vi "LIA Debugging Slow FPGA.vi"() -> ()   [LabVIEW 2018]
uses:
  <vilib>/eio/EIONode/EIONode.xnode
  <vilib>/rvi/eio/common/nirviEmuTemplateMethod_errors.vi
  <vilib>/Platform/TimedLoop/XDataNode/wakeup.ctl
  <vilib>/Platform/TimedLoop/XDataNode/XDNodeRunTimeDep.lvlib
  <vilib>/Platform/TimedLoop/XDataNode/nitl_modes.ctl
  <vilib>/Platform/TimedLoop/XDataNode/timing_clust.ctl
  <vilib>/Platform/TimedLoop/XDataNode/XDataNode.xnode
  <instrlib>/_niInstr/Basic Elements/v1/FPGA/niInstr Basic Elements v1 FPGA.lvlib
  <instrlib>/_niInstr/DSP/v1/Shared/Public/IQ Data.ctl
  <instrlib>/_niInstr/DSP/v1/Shared/niInstr DSP v1 Shared.lvlib
  <instrlib>/_niInstr/DSP/v1/FPGA/niInstr DSP v1 FPGA.lvlib
  <instrlib>/_niInstr/DSP/v1/Xnodes/Public/Frequency Shift/niInstr DSP v1 Frequency Shift FPGA.xnode
  Shared/_NI PLL IP/FPGA/NI PLL IP FPGA.lvlib
  <vilib>/rvi/FXPMathLib/FxpMul/XNode/nifxpmath_Multiplier.xnode
  <vilib>/rvi/FXPMathLib/FxpAdd/XNode/nifxpmath_Add.xnode
  <instrlib>/_niInstr/DSP/v1/FPGA/Public/Sub VIs/Frequency Shift/Frequency Shift - 2 spc.vi
  Shared/lib/fpga/Lock-In Amplifier Example FPGA.lvlib
  <instrlib>/_niInstr/Streaming/v1/Common/Stream State.ctl
  <instrlib>/_niInstr/Streaming/v1/Common/niInstr Streaming v1 Common.lvlib
  <userlib>/_NI Noise Generation IP/FPGA/NI Noise Generation IP FPGA v2.lvlib
  <vilib>/rvi/FXPMathLib/sim/FxpSim.dll
  <instrlib>/_niInstr/DSP/v1/FPGA/Public/Sub VIs/Fractional Decimator/Fractional Decimator - 1 spc - 2x oc.vi
  <userlib>/_NI Noise Generation IP/FPGA/Public/Low Level/AWGN FXP23x2.vi
  <instrlib>/_niInstr/Data Trigger/v1/Shared/Public/Edge Configuration Trigger Slope.ctl
  <instrlib>/_niInstr/Data Trigger/v1/Shared/niInstr Data Trigger v1 Shared.lvlib
  <instrlib>/_niInstr/Data Trigger/v1/Shared/Public/Edge Configuration FXP(+-,18,1).ctl
  Shared/SOS/Controls/IIR_Coeffs.ctl
panel:
  out "lock-in.fir overflow? 0":bool
  out "lock-in.prefilter fir overflow? 0":bool
  out "lock-in.fs overflow? 0":bool
  in  "lock-in.iir config prefilter 0":T1
  in  "lock-in.iir prefilter decmation 0":fxp<+,4,4>
  out "stream.overflow? 0":bool
  in  "all.clear overflow 0":bool
  in  "lock-in.fir fs prefilter 0":fxp<+,48,1>
  in  "lock-in.prefilter 0":enum16{"1x2SOS", "None", "FIR"}(ring)
  in  "lock-in.iir enable0 0":bool
  in  "lock-in.iir decimation0 0":fxp<+,4,4> format="%#_3g"
  in  "lock-in.iir config0 0":T1={"b0"=0.015777587890625, "b1"=-0.030517578125, "-a1"=1.9578399658203125, "-a2"=-0.9589080810546875}
  in  "nco.enable 0":bool=TRUE
  in  "nco.reset 0":bool
  in  "nco.frequency 0":fxp<+/-,48,0>
  in  "lock-in.fir0 fs 0":fxp<+,48,1>
  in  "lock-in.decimator0 0":enum16{"None", "CIC", "FIR", "2x4HB", "2x4SOS"}(ring)
  in  "dpll.reset 1":bool
  in  "dpll.enable 1":bool
  in  "dpll.q 1":fxp<+/-,48,0>
  in  "dpll.m 1":i8
  in  "dpll.config 1":T2
  out "dpll.vco output 1":fxp<+/-,48,0>
  in  "dpll.channel 1":i32
  in  "dpll.channel 0":i32
  out "dpll.vco output 0":fxp<+/-,48,0>
  in  "dpll.config 0":T2
  in  "dpll.m 0":i8
  in  "dpll.q 0":fxp<+/-,48,0>
  in  "dpll.enable 0":bool
  in  "dpll.reset 0":bool
  in  "lock-in.enable 3":bool
  in  "lock-in.enable 2":bool
  in  "lock-in.enable 1":bool
  in  "lock-in.carrier 3":fxp<+/-,48,0>
  in  "lock-in.carrier 2":fxp<+/-,48,0>
  in  "lock-in.enable 0":bool
  in  "lock-in.channel select 3":i32
  in  "lock-in.carrier select 3":i32
  in  "lock-in.cic config valid 3":bool
  in  "lock-in.cic config 3":cluster{"factor":fxp<+,16,16>, "shift":i16}
  in  "lock-in.reset 3":bool
  out "stream.state 3":T4 caption="stream.state 0"
  out "stream.samples transferred 3":u64 caption="stream.samples transferred 0"
  out "stream.metadata 3":u64 caption="stream.metadata 0"
  in  "stream.num samples 3":u64 caption="stream.num samples 0"
  in  "stream.request state 3":T4 caption="stream.request state 0"
  in  "lock-in.channel select 2":i32
  in  "lock-in.carrier select 2":i32
  in  "lock-in.cic config valid 2":bool
  in  "lock-in.cic config 2":cluster{"factor":fxp<+,16,16>, "shift":i16}
  in  "lock-in.reset 2":bool
  out "stream.state 2":T4 caption="stream.state 0"
  out "stream.samples transferred 2":u64 caption="stream.samples transferred 0"
  out "stream.metadata 2":u64 caption="stream.metadata 0"
  in  "stream.num samples 2":u64 caption="stream.num samples 0"
  in  "stream.request state 2":T4 caption="stream.request state 0"
  out "pll.vco output 0":fxp<+/-,48,0>
  out "pll.vco output 1":fxp<+/-,48,0>
  out "stream.metadata 4":u64 caption="stream.metadata 0"
  out "stream.samples transferred 4":u64 caption="stream.samples transferred 0"
  out "stream.state 4":T4 caption="stream.state 0"
  in  "stream.request state 4":T4 caption="stream.request state 0"
  in  "stream.num samples 4":u64 caption="stream.num samples 0"
  in  "preview.channel select":i32
  in  "ao.reset 3":bool
  in  "ao.carrier 2":fxp<+/-,48,0>=0.010000000000001563
  in  "ao.level 2":fxp<+/-,18,1>
  in  "ao.reset 2":bool
  in  "ao.carrier 1":fxp<+/-,48,0>=0.010000000000001563
  in  "ao.level 1":fxp<+/-,18,1>
  in  "ao.reset 1":bool
  in  "ao.reset 0":bool
  in  "ao.carrier 0":fxp<+/-,48,0>=0.010000000000001563
  in  "ao.level 0":fxp<+/-,18,1>
  in  "lock-in.channel select 1":i32
  in  "lock-in.channel select 0":i32
  in  "stream.request state 1":T4 caption="stream.request state 0"
  in  "stream.num samples 1":u64 caption="stream.num samples 0"
  out "stream.metadata 1":u64 caption="stream.metadata 0"
  out "stream.samples transferred 1":u64 caption="stream.samples transferred 0"
  out "stream.state 1":T4 caption="stream.state 0"
  in  "lock-in.reset 1":bool
  in  "lock-in.cic config 1":cluster{"factor":fxp<+,16,16>, "shift":i16}
  in  "lock-in.cic config valid 1":bool
  in  "lock-in.carrier select 1":i32
  in  "lock-in.carrier select 0":i32
  in  "lock-in.cic config valid 0":bool
  in  "lock-in.cic config 0":cluster{"factor":fxp<+,16,16>, "shift":i16}
  in  "lock-in.reset 0":bool
  in  "lock-in.carrier 1":fxp<+/-,48,0>
  in  "lock-in.carrier 0":fxp<+/-,48,0>
  in  "ao.level 3":fxp<+/-,18,1>
  in  "pll.channel 1":i32
  in  "pll.reset 1":bool
  in  "pll.enable 1":bool
  in  "pll.config 1":T5={"quiescent frequency"=0.10000000000000142, "compensation"=0.0, "psd gain"=-18, "loop filter"={"order"=4, "cutoff"=6}}
  in  "pll.channel 0":i32
  in  "ao.noise gain 3":fxp<+,18,1>=0.01000213623046875
  in  "ao.carrier 3":fxp<+/-,48,0>=0.010000000000001563
  in  "ao.noise seeds 3":fxp<+,23,23>[](array[numeric])=[1.0, 12323.0]
  in  "pll.reset 0":bool
  in  "pll.enable 0":bool
  in  "stream.request state 0":T4
  in  "stream.num samples 0":u64
  out "stream.metadata 0":u64
  out "stream.samples transferred 0":u64
  out "stream.state 0":T4
  in  "pll.config 0":T5={"quiescent frequency"=0.10000000000000142, "compensation"=0.0, "psd gain"=-18, "loop filter"={"order"=4, "cutoff"=6}}
  out "IO Module\\InitDone":bool
  out "IO Module\\User Error":u32
  in  "IO Module\\User Command":u32
  in  "IO Module\\User Command Valid":bool
  out "IO Module\\User Command Ready":bool
  in  "IO Module\\User Command Arg 0":u32
  in  "IO Module\\User Command Arg 1":u32
  out "IO Module\\User Command Error":u16
  out "IO Module\\User Command Return":u32
  out "IO Module\\User Command Return Valid":bool
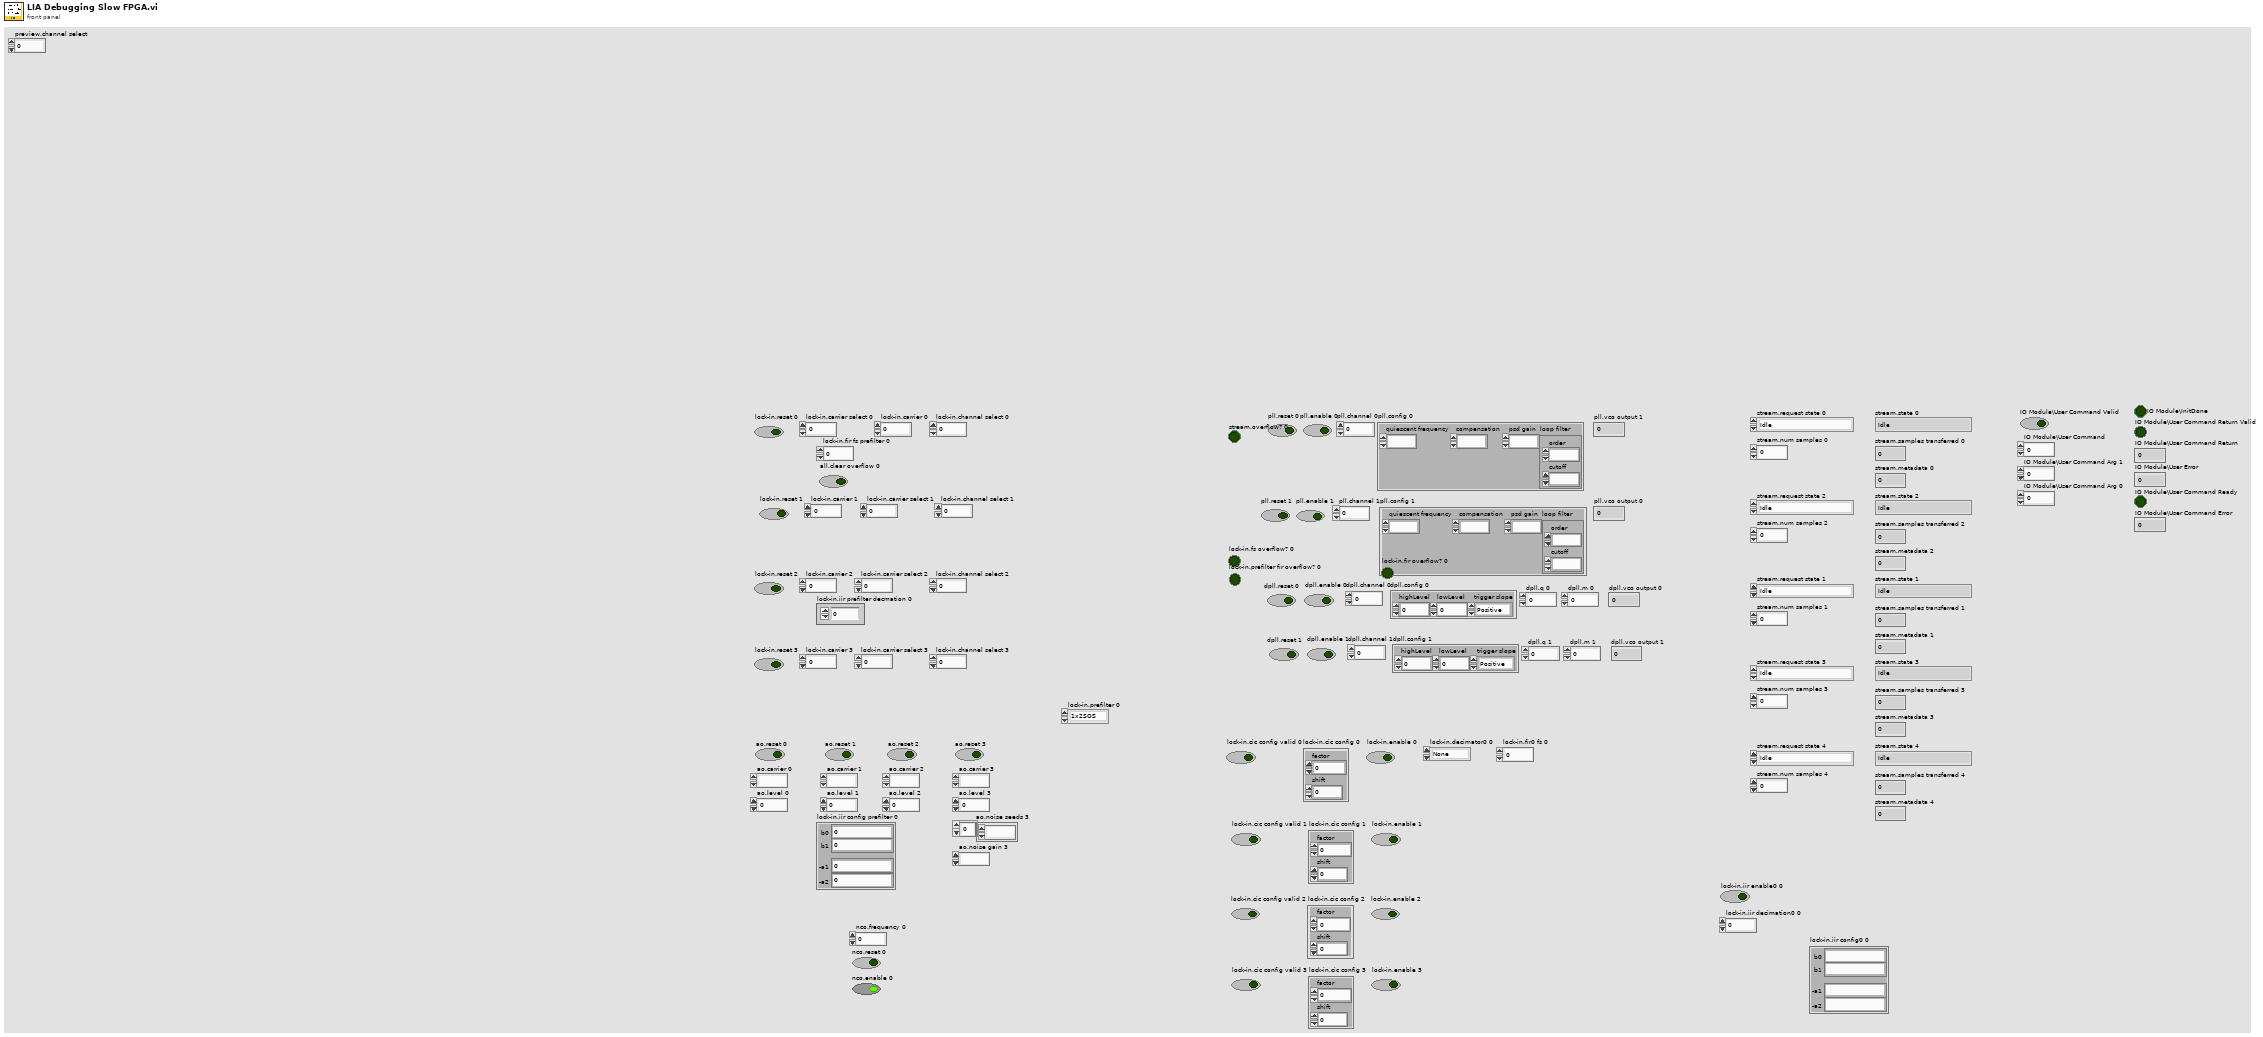
[diagram p1: front panel]
types:
  T1 = typedef "IIR_Coeffs.ctl" = cluster{"b0":fxp<+/-,18,2>, "b1":fxp<+/-,18,2>, "-a1":fxp<+/-,18,2>, "-a2":fxp<+/-,18,2>}
  T2 = typedef "niInstr Data Trigger v1 Shared.lvlib/Edge Configuration FXP(+-,18,1).ctl" = cluster{"highLevel":fxp<+/-,18,1>, "lowLevel":fxp<+/-,18,1>, "trigger slope":T3}
  T3 = typedef "niInstr Data Trigger v1 Shared.lvlib/Edge Configuration Trigger Slope.ctl" = enum8{"Positive", "Negative"}
  T4 = typedef "niInstr Streaming v1 Common.lvlib/Stream State.ctl" = enum8{"Idle", "Finite Transfer", "Continuous", "Done", "Error", "Not Ready", "Cancel"}
  T5 = cluster{"quiescent frequency":fxp<+/-,48,0>, "compensation":fxp<+/-,18,3>, "psd gain":i16, "loop filter":cluster{"order":i32, "cutoff":i8}}
  T6 = typedef "XDNodeRunTimeDep.lvlib/timing_clust.ctl" = cluster{"Expected End [f-1]":u64, "Actual End [f-1]":u64, "Finished Late? [f-1]":bool, "Expected End [i-1]":u64, "Actual End [i-1]":u64, "Finished Late? [i-1]":bool, "Expected Start [i]":u64, "Actual Start [i]":u64, "Expected Start [f]":u64, "Actual Start [f]":u64, "Source Name":string, "Structure Name":string, "Period":i64, "Deadline":i64, "Offset":i64, "Start":i64, "Priority":i32, "Timeout":i32, "Mode":T7, "Wakeup Reason":T8, "Error":errorcluster, "Source Type":string, "Secondary Source Type":string, "Global End Time":u64, "Global Start Time":u64, "Frame Duration":u64, "Iteration Duration":u64, "Assigned CPU":i32, "I/O Scan Engine Mode":u32}
  T7 = typedef "XDNodeRunTimeDep.lvlib/nitl_modes.ctl" = enum32{"No Change", "Process missed periods, maintain original phase", "Discard missed periods, maintain original phase", "Process missed periods, ignore original phase", "Discard missed periods, ignore original phase"}
  T8 = typedef "XDNodeRunTimeDep.lvlib/wakeup.ctl" = enum32{"Normal", "Aborted", "Asynchronous wakeup", "Timing source error", "Timed loop error", "Timeout"}
  T9 = cluster{"stream.num samples 0":u64, "stream.request state 0":T4, "stream.index 0":i16}
  T10 = typedef "niInstr DSP v1 Shared.lvlib/IQ Data.ctl" = cluster{"I":fxp<+/-,18,1>, "Q":fxp<+/-,18,1>, "overflow":bool}
  T11 = cluster{"stream.metadata 0":u64, "stream.samples transferred 0":u64, "stream.state 0":T4}
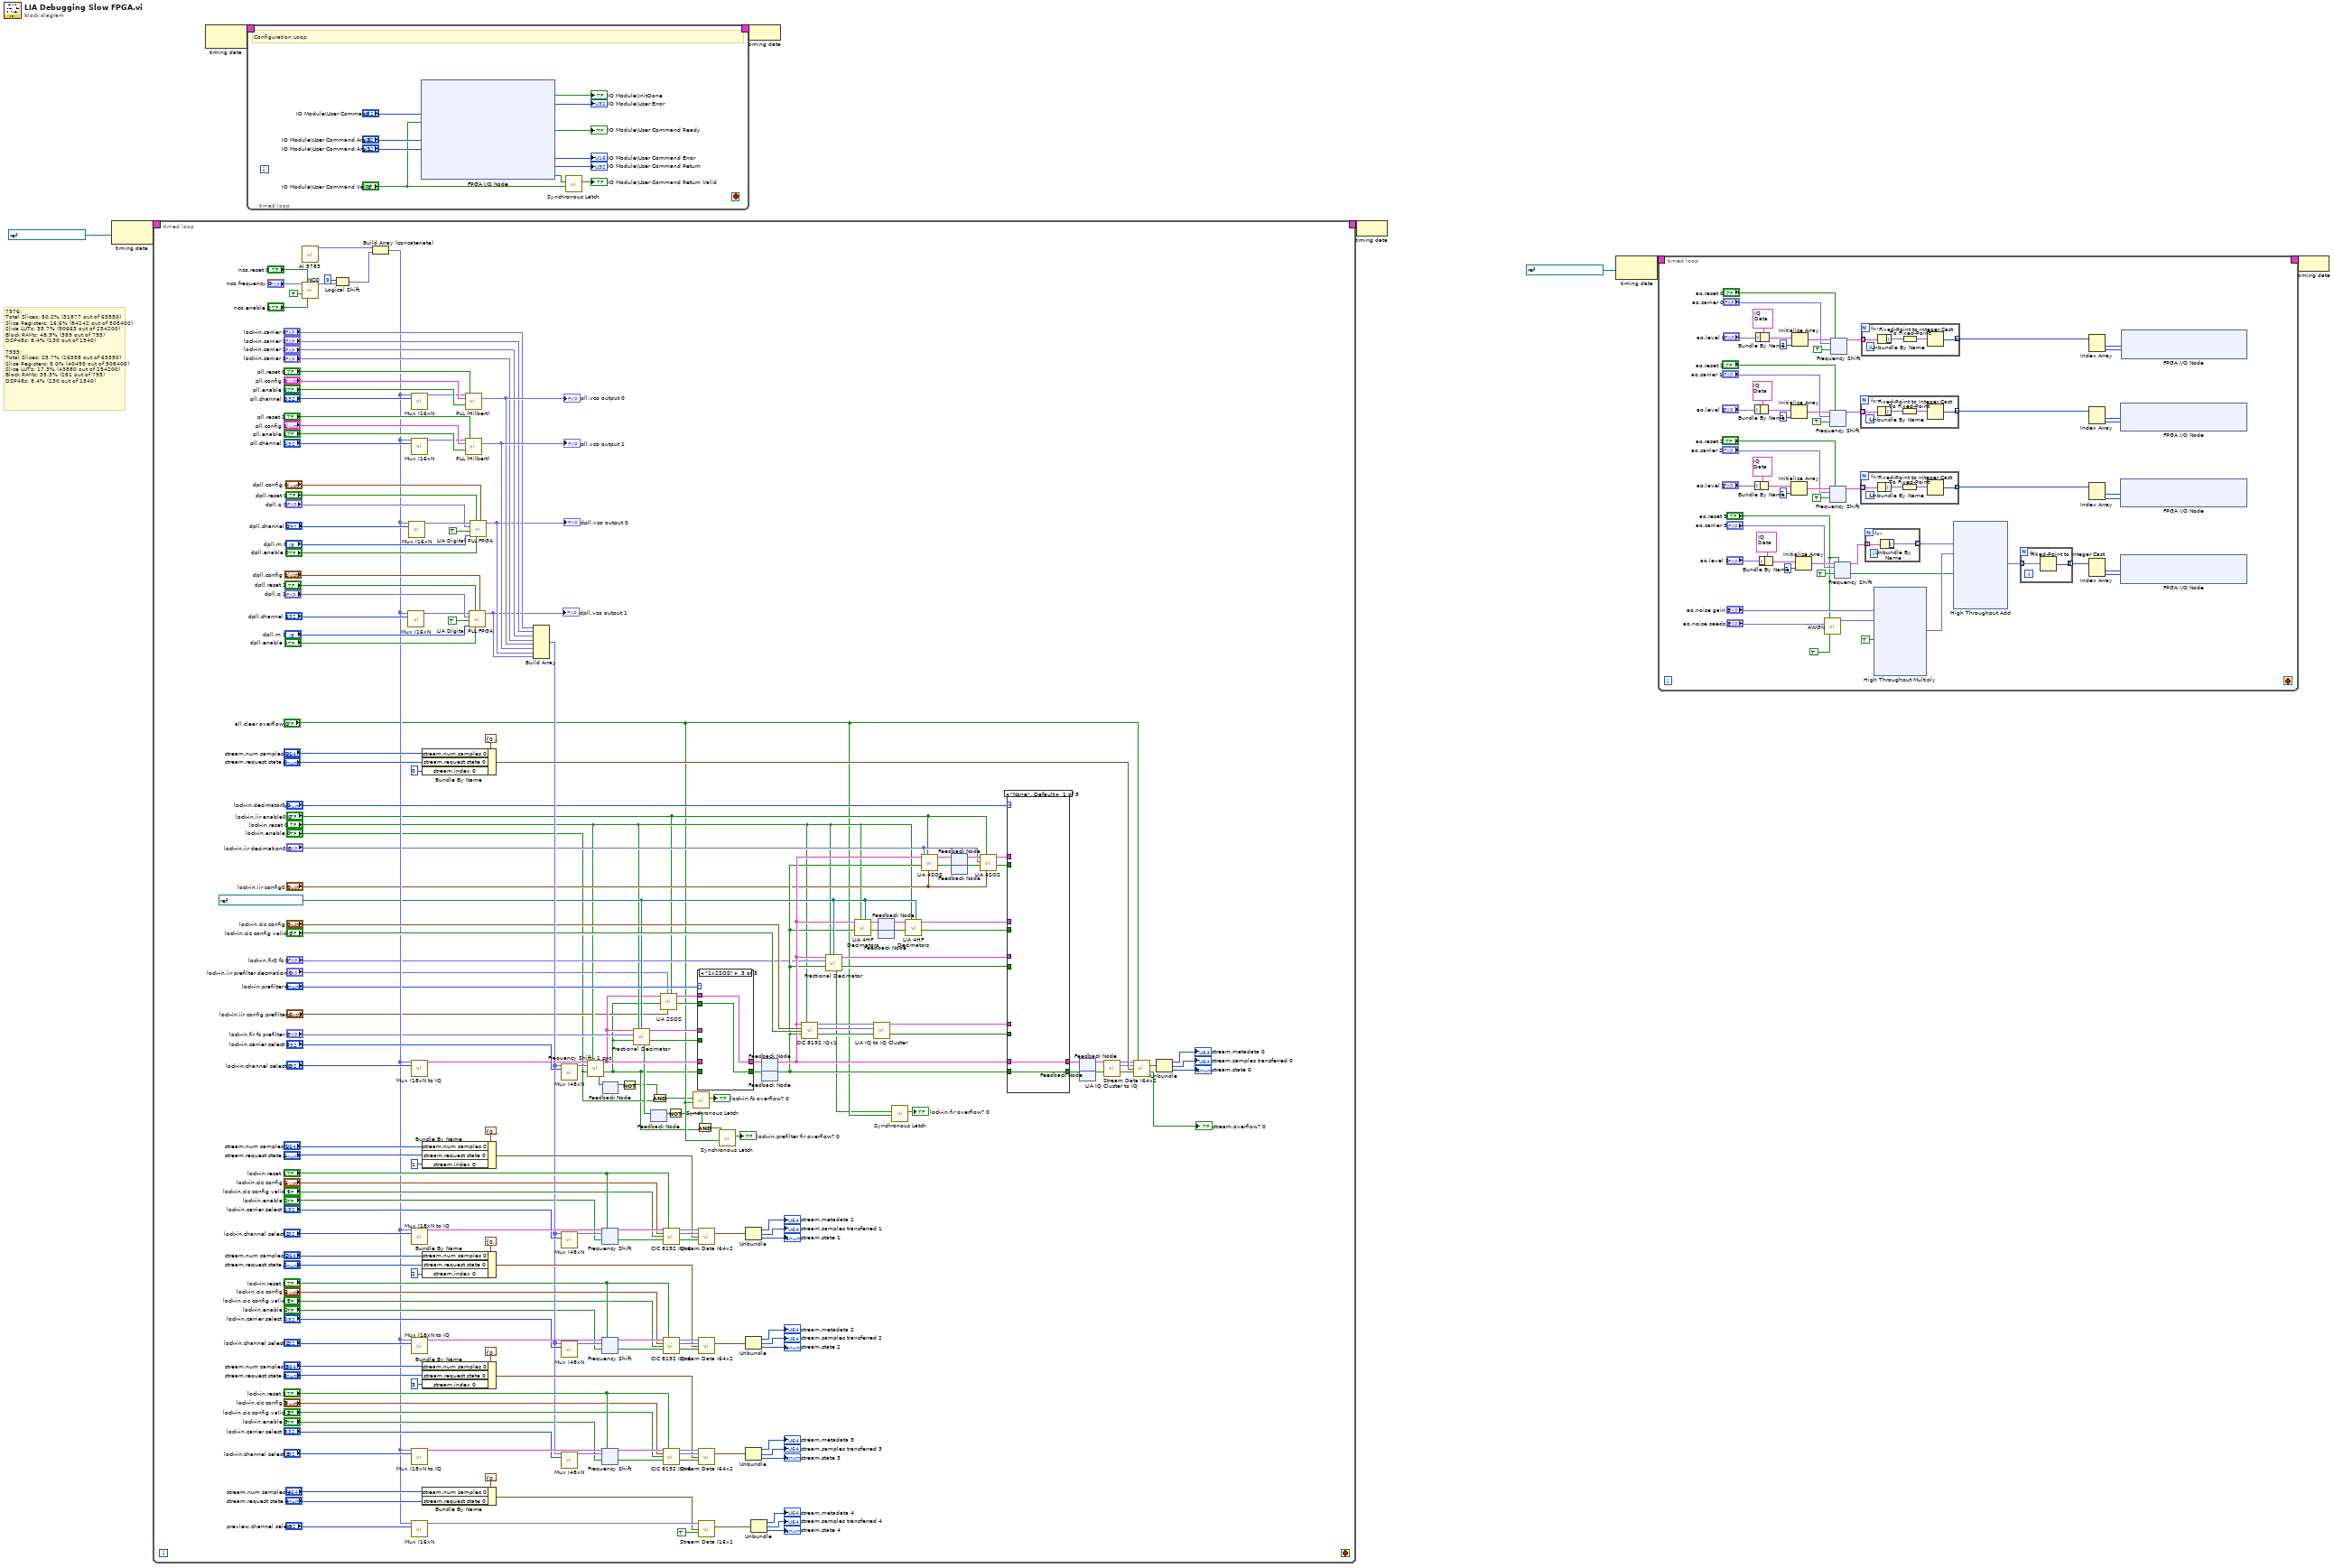
[diagram p0: block diagram]
diagram:
  # "7976:\nTotal Slices: 50.2% (31877 out of 63550)\nSlice Registers: 16.6% (84242 out of 508400)\nSlice LUTs: 35.7% (90663 out of 254200)\nBlock RAMs: 48.9% (389 out of 795)\nDSP48s: 8.4% (130 out of 1540)\n\n7935:\nTotal Slices: 25.7% (16358 out of 63550)\nSlice Registers: 8.0% (40499 out of 508400)\nSlice LUTs: 17.3% (43880 out of 254200)\nBlock RAMs: 35.3% (281 out of 795)\nDSP48s: 8.4% (130 out of 1540)"
  n1 = node-c288(refnum<k21> "IO Module\\Data Clock" ("Source Name")) -> (w8:T6)
  n2 = timed-loop {
    timing: w8 -> [_]
    timing-out: [_] -> w7
    stop <- _ stop-if-true
    w50 = refnum<k21> "IO Module\\Data Clock 2x" ("clock x 2")
    n3 = call "AI 5783.vi"() -> ("i18x1"=w82:fxp<+/-,18,1>[])  [unwired: 14 in, 1 out]
    n4 = call <instrlib>:"NCO.vi"("frequency"="nco.frequency 0", "reset"="nco.reset 0", "input valid"=TRUE, "enable (T)"="nco.enable 0") -> ("cosine out"=w65:fxp<+/-,18,1>)  [unwired: 9 in, 2 out]
    n5 = Logical Shift(y=i16 0, x=w65) -> (x << y=w66:fxp<+/-,18,1>)
    n6 = Build Array (concatenate)(w82, w66) -> (w76:fxp<+/-,18,1>[])
    n7 = call "Mux I16xN.vi"("i16xn in"=w76, "index"="dpll.channel 1") -> ("i16 out"=w85:fxp<+/-,18,1>)  [unwired: 12 in, 1 out]
    n8 = call "Mux I16xN.vi"("i16xn in"=w76, "index"="dpll.channel 0") -> ("i16 out"=w97:fxp<+/-,18,1>)  [unwired: 12 in, 1 out]
    n9 = call "Mux I16xN.vi"("i16xn in"=w76, "index"="pll.channel 0") -> ("i16 out"=w201:fxp<+/-,18,1>)  [unwired: 12 in, 1 out]
    n10 = call "Mux I16xN.vi"("i16xn in"=w76, "index"="pll.channel 1") -> ("i16 out"=w195:fxp<+/-,18,1>)  [unwired: 12 in, 1 out]
    n11 = call "Mux I18xN to IQ.vi"("i16xn in"=w76, "index"="lock-in.channel select 0") -> ("output"=w61:T10)  [unwired: 12 in, 1 out]
    n12 = call "Mux I18xN to IQ.vi"("i16xn in"=w76, "index"="lock-in.channel select 1") -> ("output"=w183:T10)  [unwired: 12 in, 1 out]
    n13 = call "Mux I18xN to IQ.vi"("i16xn in"=w76, "index"="lock-in.channel select 2") -> ("output"=w149:T10)  [unwired: 12 in, 1 out]
    n14 = call "Mux I18xN to IQ.vi"("i16xn in"=w76, "index"="lock-in.channel select 3") -> ("output"=w128:T10)  [unwired: 12 in, 1 out]
    n15 = call "Mux I16xN.vi"("i16xn in"=w76, "index"="preview.channel select") -> ("i16 out"=w157:fxp<+/-,18,1>)  [unwired: 12 in, 1 out]
    n16 = Bundle By Name(cluster=T9 {"stream.num samples 0"=0, "stream.request state 0"=enum."Idle", "stream.index 0"=0} ("config"), "stream.num samples 0"="stream.num samples 0", "stream.request state 0"="stream.request state 0", "stream.index 0"=i16 0) -> (w186:T9)
    n17 = Bundle By Name(cluster=T9 {"stream.num samples 0"=0, "stream.request state 0"=enum."Idle", "stream.index 0"=0} ("config"), "stream.num samples 0"="stream.num samples 1", "stream.request state 0"="stream.request state 1", "stream.index 0"=i16 1) -> (w165:T9)
    n18 = Bundle By Name(cluster=T9 {"stream.num samples 0"=0, "stream.request state 0"=enum."Idle", "stream.index 0"=0} ("config"), "stream.num samples 0"="stream.num samples 2", "stream.request state 0"="stream.request state 2", "stream.index 0"=i16 2) -> (w131:T9)
    n19 = Bundle By Name(cluster=T9 {"stream.num samples 0"=0, "stream.request state 0"=enum."Idle", "stream.index 0"=0} ("config"), "stream.num samples 0"="stream.num samples 3", "stream.request state 0"="stream.request state 3", "stream.index 0"=i16 3) -> (w110:T9)
    n20 = Bundle By Name(cluster=T9 {"stream.num samples 0"=0, "stream.request state 0"=enum."Idle", "stream.index 0"=0} ("config"), "stream.num samples 0"="stream.num samples 4", "stream.request state 0"="stream.request state 4") -> (w153:T9)
    n21 = call "PLL (Hilbert).vi"("input"=w201, "reset"="pll.reset 0", "config"="pll.config 0", "enable"="pll.enable 0") -> ("output"=w150:fxp<+/-,48,0>)  [unwired: 11 in]
    "pll.vco output 0" <- w150
    n22 = call "PLL (Hilbert).vi"("input"=w195, "reset"="pll.reset 1", "config"="pll.config 1", "enable"="pll.enable 1") -> ("output"=w151:fxp<+/-,48,0>)  [unwired: 11 in]
    "pll.vco output 1" <- w151
    n23 = call "LIA Digital PLL FPGA.vi"("configuration"="dpll.config 1", "arm"="dpll.enable 1", "reset"="dpll.reset 1", "m"="dpll.m 1", "input valid"=TRUE, "q"="dpll.q 1", "I"=w85) -> ("frequency shift"=w81:fxp<+/-,48,0>)  [unwired: 1 in, 3 out]
    "dpll.vco output 1" <- w81
    n24 = call "LIA Digital PLL FPGA.vi"("configuration"="dpll.config 0", "arm"="dpll.enable 0", "reset"="dpll.reset 0", "m"="dpll.m 0", "input valid"=TRUE, "q"="dpll.q 0", "I"=w97) -> ("frequency shift"=w92:fxp<+/-,48,0>)  [unwired: 1 in, 3 out]
    "dpll.vco output 0" <- w92
    n25 = Build Array("lock-in.carrier 0", "lock-in.carrier 1", "lock-in.carrier 2", "lock-in.carrier 3", w150, w151, w92, w81) -> (w107:fxp<+/-,48,0>[])
    n26 = call "Mux I48xN.vi"("i48xn in"=w107, "index"="lock-in.carrier select 0") -> ("i48 out"=w60:fxp<+/-,48,0>)  [unwired: 13 in]
    n27 = call "Mux I48xN.vi"("i48xn in"=w107, "index"="lock-in.carrier select 1") -> ("i48 out"=w182:fxp<+/-,48,0>)  [unwired: 13 in]
    n28 = call "Mux I48xN.vi"("i48xn in"=w107, "index"="lock-in.carrier select 2") -> ("i48 out"=w148:fxp<+/-,48,0>)  [unwired: 13 in]
    n29 = call "Mux I48xN.vi"("i48xn in"=w107, "index"="lock-in.carrier select 3") -> ("i48 out"=w127:fxp<+/-,48,0>)  [unwired: 13 in]
    n30 = call <instrlib>:"Frequency Shift - 1 spc.vi"("data in"=w61, "reset"="lock-in.reset 0", "frequency shift"=w60, "input valid"="lock-in.enable 0") -> ("data out"=w29:T10, "output valid"=w12:bool, "ready for input"=w23:bool)  [unwired: 8 in, 1 out]
    n31 = xnode "Frequency Shift"("data in"=w183, "reset"="lock-in.reset 1", "frequency shift"=w182, "input valid"="lock-in.enable 1") -> ("data out"=w181:T10, "output valid"=w180:bool)  [unwired: 2 in, 1 out]
    n32 = xnode "Frequency Shift"("data in"=w149, "reset"="lock-in.reset 2", "frequency shift"=w148, "input valid"="lock-in.enable 2") -> ("data out"=w147:T10, "output valid"=w146:bool)  [unwired: 2 in, 1 out]
    n33 = xnode "Frequency Shift"("data in"=w128, "reset"="lock-in.reset 3", "frequency shift"=w127, "input valid"="lock-in.enable 3") -> ("data out"=w126:T10, "output valid"=w125:bool)  [unwired: 2 in, 1 out]
    n34 = feedback-in #1(w23) -> ()
    n35 = feedback #1() -> (w14:bool)  [unwired: 1 in]
    n36 = Not(x=w14) -> (.not. x?=w11:bool)
    n37 = call-poly <instrlib>:"Fractional Decimator.vi"("data in"=w29, "reset"="lock-in.reset 0", "clock x 2"=w50, "output sample rate"="lock-in.fir fs prefilter 0", "input valid"=w12) -> ("data out"=w46:T10, "output valid"=w45:bool, "ready for input"=w20:bool)  [unwired: 8 in]
    n38 = feedback-in #2(w20) -> ()
    n39 = feedback #2() -> (w10:bool)  [unwired: 1 in]
    n40 = And(x=w11, y="lock-in.enable 0") -> (x .and. y?=w16:bool)
    n41 = call "LIA 2SOS.vi"("lock-in.iir enable0 0"="lock-in.iir enable0 0", "lock-in.iir config0 0"="lock-in.iir config prefilter 0", "lock-in.iir decimation0 0"="lock-in.iir prefilter decmation 0", "input valid"=w12, "IQ_Data_In"=w29) -> ("output valid"=w25:bool, "IQ_Data_Out"=w26:T10)  [unwired: 5 in]
    n42 = call "CIC 8192 IQx1.vi"("data"=w181, "reset"="lock-in.reset 1", "config"="lock-in.cic config 1", "config valid"="lock-in.cic config valid 1", "input valid"=w180) -> ("i out"=w176:fxp<+/-,64,1>, "q out"=w175:fxp<+/-,64,1>, "output valid"=w174:bool)  [unwired: 8 in]
    n43 = call "CIC 8192 IQx1.vi"("data"=w147, "reset"="lock-in.reset 2", "config"="lock-in.cic config 2", "config valid"="lock-in.cic config valid 2", "input valid"=w146) -> ("i out"=w142:fxp<+/-,64,1>, "q out"=w141:fxp<+/-,64,1>, "output valid"=w140:bool)  [unwired: 8 in]
    n44 = call "CIC 8192 IQx1.vi"("data"=w126, "reset"="lock-in.reset 3", "config"="lock-in.cic config 3", "config valid"="lock-in.cic config valid 3", "input valid"=w125) -> ("i out"=w121:fxp<+/-,64,1>, "q out"=w120:fxp<+/-,64,1>, "output valid"=w119:bool)  [unwired: 8 in]
    n45 = Not(x=w10) -> (.not. x?=w9:bool)
    n46 = call <instrlib>:"Synchronous Latch.vi"("clear"="all.clear overflow 0", "set"=w16) -> ("out"=→"lock-in.fs overflow? 0":bool)  [unwired: 9 in]
    n47 = And(x=w9, y=w12) -> (x .and. y?=w13:bool)
    n48 = case shown="\"1x2SOS\"" "lock-in.prefilter 0" {
      tunnel: w29 -> [w206 _ _]
      tunnel: w12 -> [w205 _ _]
      tunnel: [w206 w208 w210] -> w47
      tunnel: [w205 w207 w209] -> w39
      tunnel: w46 -> [_ w208 _]
      tunnel: w45 -> [_ w207 _]
      tunnel: w26 -> [_ _ w210]
      tunnel: w25 -> [_ _ w209]
      frame "None", Default {
      }
      frame "FIR" {
      }
      frame "1x2SOS" {
      }
    }
    n49 = call "Stream Data I64x2.vi"("i in"=w176, "q in"=w175, "config"=w165, "input valid"=w174) -> ("status"=w173:T11)  [unwired: 10 in, 1 out]
    n50 = call "Stream Data I64x2.vi"("i in"=w142, "q in"=w141, "config"=w131, "input valid"=w140) -> ("status"=w139:T11)  [unwired: 10 in, 1 out]
    n51 = call "Stream Data I64x2.vi"("i in"=w121, "q in"=w120, "config"=w110, "input valid"=w119) -> ("status"=w118:T11)  [unwired: 10 in, 1 out]
    n52 = call "Stream Data I16x1.vi"("i in"=w157, "config"=w153, "input valid"=TRUE) -> ("status"=w159:T11)  [unwired: 12 in]
    n53 = call <instrlib>:"Synchronous Latch.vi"("clear"="all.clear overflow 0", "set"=w13) -> ("out"=→"lock-in.prefilter fir overflow? 0":bool)  [unwired: 9 in]
    n54 = Unbundle(w173) -> ("stream.metadata 0"=→"stream.metadata 1":u64, "stream.samples transferred 0"=→"stream.samples transferred 1":u64, "stream.state 0"=→"stream.state 1":T4)
    n55 = Unbundle(w139) -> ("stream.metadata 0"=→"stream.metadata 2":u64, "stream.samples transferred 0"=→"stream.samples transferred 2":u64, "stream.state 0"=→"stream.state 2":T4)
    n56 = Unbundle(w118) -> ("stream.metadata 0"=→"stream.metadata 3":u64, "stream.samples transferred 0"=→"stream.samples transferred 3":u64, "stream.state 0"=→"stream.state 3":T4)
    n57 = Unbundle(w159) -> ("stream.metadata 0"=→"stream.metadata 4":u64, "stream.samples transferred 0"=→"stream.samples transferred 4":u64, "stream.state 0"=→"stream.state 4":T4)
    n58 = feedback-in #3(w47) -> ()
    n59 = feedback #3() -> (w40:T10)  [unwired: 1 in]
    n60 = feedback #4() -> (w38:bool)  [unwired: 1 in]
    n61 = feedback-in #4(w39) -> ()
    n62 = call "CIC 8192 IQx1.vi"("data"=w40, "reset"="lock-in.reset 0", "config"="lock-in.cic config 0", "config valid"="lock-in.cic config valid 0", "input valid"=w38) -> ("i out"=w69:fxp<+/-,64,1>, "q out"=w68:fxp<+/-,64,1>, "output valid"=w77:bool)  [unwired: 8 in]
    n63 = call-poly <instrlib>:"Fractional Decimator.vi"("data in"=w40, "reset"="lock-in.reset 0", "clock x 2"=w50, "output sample rate"="lock-in.fir0 fs 0", "input valid"=w38) -> ("data out"=w70:T10, "output valid"=w71:bool, "ready for input"=w17:bool)  [unwired: 8 in]
    n64 = call "LIA 4HF Decimators.vi"("clock x 2"=w50, "reset"="lock-in.reset 0", "input valid"=w38, "data in"=w40) -> ("output valid"=w58:bool, "data out"=w59:T10)  [unwired: 6 in]
    n65 = call "LIA IQ to IQ Cluster.vi"("i in"=w69, "q in"=w68) -> ("data out"=w67:T10)  [unwired: 13 in]
    n66 = feedback-in #5(w59) -> ()
    n67 = feedback #5() -> (w35:T10)  [unwired: 1 in]
    n68 = feedback-in #6(w58) -> ()
    n69 = feedback #6() -> (w34:bool)  [unwired: 1 in]
    n70 = call <instrlib>:"Synchronous Latch.vi"("clear"="all.clear overflow 0", "set"=w17) -> ("out"=→"lock-in.fir overflow? 0":bool)  [unwired: 9 in]
    n71 = call "LIA 4HF Decimators.vi"("clock x 2"=w50, "reset"="lock-in.reset 0", "input valid"=w34, "data in"=w35) -> ("output valid"=w57:bool, "data out"=w56:T10)  [unwired: 6 in]
    n72 = call "LIA 4SOS.vi"("lock-in.iir config0 0"="lock-in.iir config0 0", "lock-in.iir enable0 0"="lock-in.iir enable0 0", "input valid"=w38, "lock-in.iir decimation0 0"="lock-in.iir decimation0 0", "IQ_Data_In"=w40) -> ("output valid"=w53:bool, "IQ_Data_Out"=w54:T10)  [unwired: 5 in]
    n73 = feedback-in #7(w54) -> ()
    n74 = feedback #7() -> (w37:T10)  [unwired: 1 in]
    n75 = feedback-in #8(w53) -> ()
    n76 = feedback #8() -> (w36:bool)  [unwired: 1 in]
    n77 = call "LIA 4SOS.vi"("lock-in.iir config0 0"="lock-in.iir config0 0", "lock-in.iir enable0 0"="lock-in.iir enable0 0", "input valid"=w36, "lock-in.iir decimation0 0"="lock-in.iir decimation0 0", "IQ_Data_In"=w37) -> ("output valid"=w51:bool, "IQ_Data_Out"=w52:T10)  [unwired: 5 in]
    n78 = case shown="\"None\", Default" "lock-in.decimator0 0" {
      tunnel: [w212 w214 w216 w218 w219] -> w62
      tunnel: w77 -> [_ w214 _ _ _]
      tunnel: w71 -> [_ _ w216 _ _]
      tunnel: w38 -> [w212 _ _ _ _]
      tunnel: w70 -> [_ _ w215 _ _]
      tunnel: w40 -> [w211 _ _ _ _]
      tunnel: w56 -> [_ _ _ w217 _]
      tunnel: w57 -> [_ _ _ w218 _]
      tunnel: [w211 w213 w215 w217 w220] -> w63
      tunnel: w67 -> [_ w213 _ _ _]
      tunnel: w52 -> [_ _ _ _ w220]
      tunnel: w51 -> [_ _ _ _ w219]
      frame "None", Default {
      }
      frame "CIC" {
      }
      frame "FIR" {
      }
      frame "2x4HB" {
      }
      frame "2x4SOS" {
      }
    }
    n79 = feedback #9() -> (w44:T10)  [unwired: 1 in]
    n80 = feedback-in #9(w63) -> ()
    n81 = feedback #10() -> (w55:bool)  [unwired: 1 in]
    n82 = feedback-in #10(w62) -> ()
    n83 = call "LIA IQ Cluster to IQ.vi"("data in"=w44) -> ("i in"=w43:fxp<+/-,64,1>, "q in"=w42:fxp<+/-,64,1>)  [unwired: 13 in]
    n84 = call "Stream Data I64x2.vi"("i in"=w43, "clear overflow"="all.clear overflow 0", "q in"=w42, "config"=w186, "input valid"=w55) -> ("status"=w194:T11, "overflow?"=→"stream.overflow? 0":bool)  [unwired: 9 in]
    n85 = Unbundle(w194) -> ("stream.metadata 0"=→"stream.metadata 0":u64, "stream.samples transferred 0"=→"stream.samples transferred 0":u64, "stream.state 0"=→"stream.state 0":T4)
  }
  n86 = node-c288() -> (w2:T6)  [unwired: 1 in]
  n87 = timed-loop {
    timing: w2 -> [_]
    timing-out: [_] -> w1
    stop <- _ stop-if-true
    # "Configuration Loop"
    n88 = xnode "FPGA I/O Node"("IO Module\\User Command"="IO Module\\User Command", "IO Module\\User Command Valid"="IO Module\\User Command Valid", "IO Module\\User Command Arg 0"="IO Module\\User Command Arg 0", "IO Module\\User Command Arg 1"="IO Module\\User Command Arg 1") -> ("IO Module\\InitDone"=→"IO Module\\InitDone":bool, "IO Module\\Clip Error Code"=→"IO Module\\User Error":u32, "IO Module\\User Command Ready"=→"IO Module\\User Command Ready":bool, "IO Module\\User Command Error"=→"IO Module\\User Command Error":u16, "IO Module\\User Command Return"=→"IO Module\\User Command Return":u32, "IO Module\\User Command Return Valid"=w251:bool)  [unwired: 10 in, 10 out]
    n89 = call <instrlib>:"Synchronous Latch.vi"("clear"="IO Module\\User Command Valid", "set"=w251) -> ("out"=→"IO Module\\User Command Return Valid":bool)  [unwired: 9 in]
  }
  n90 = node-c288(w1) -> ()
  n91 = node-c288(w7) -> ()
  n92 = node-c288(refnum<k21> "IO Module\\Data Clock" ("Source Name")) -> (w5:T6)
  n93 = timed-loop {
    timing: w5 -> [_]
    timing-out: [_] -> w4
    stop <- _ stop-if-true
    n94 = Bundle By Name(cluster=T10 {"I"=0.0, "Q"=0.0, "overflow"=FALSE} ("output"), "I"="ao.level 1") -> (w284:T10)
    n95 = Bundle By Name(cluster=T10 {"I"=0.0, "Q"=0.0, "overflow"=FALSE} ("output"), "I"="ao.level 2") -> (w274:T10)
    n96 = Bundle By Name(cluster=T10 {"I"=0.0, "Q"=0.0, "overflow"=FALSE} ("output"), "I"="ao.level 0") -> (w299:T10)
    n97 = Bundle By Name(cluster=T10 {"I"=0.0, "Q"=0.0, "overflow"=FALSE} ("output"), "I"="ao.level 3") -> (w308:T10)
    n98 = Initialize Array(w284, 2 ("dimension size")) -> (w280:T10[])
    n99 = Initialize Array(w274, 2 ("dimension size")) -> (w278:T10[])
    n100 = Initialize Array(w299, 2 ("dimension size")) -> (w303:T10[])
    n101 = Initialize Array(w308, 2 ("dimension size")) -> (w304:T10[])
    n102 = call-poly <userlib>:"AWGN.vi"("reset"="ao.reset 3", "seeds"="ao.noise seeds 3", "ready"=TRUE) -> ("output 0"=w311:fxp<+/-,23,4>[])  [unwired: 10 in, 2 out]
    n103 = xnode "Frequency Shift"("data in"=w280, "reset"="ao.reset 1", "frequency shift"="ao.carrier 1", "input valid"=TRUE) -> ("data out"=w288:T10[])  [unwired: 2 in, 2 out]
    n104 = xnode "Frequency Shift"("data in"=w278, "reset"="ao.reset 2", "frequency shift"="ao.carrier 2", "input valid"=TRUE) -> ("data out"=w270:T10[])  [unwired: 2 in, 2 out]
    n105 = xnode "Frequency Shift"("data in"=w303, "reset"="ao.reset 0", "frequency shift"="ao.carrier 0", "input valid"=TRUE) -> ("data out"=w295:T10[])  [unwired: 2 in, 2 out]
    n106 = xnode "Frequency Shift"("data in"=w304, "reset"="ao.reset 3", "frequency shift"="ao.carrier 3", "input valid"=TRUE) -> ("data out"=w319:T10[], "output valid"=w316:bool)  [unwired: 2 in, 1 out]
    n107 = for {
      tunnel: w288 -> [w335] mode=indexing
      tunnel: [w336] -> w289 mode=indexing
      n108 = Unbundle By Name(w335) -> ("I"=w334:fxp<+/-,18,1>)
      n109 = To Fixed-Point(number=w334) -> (fixed-point=w333:fxp<+/-,16,1>)  [unwired: 1 in]
      n110 = Fixed-Point to Integer Cast(1:w333) -> (0:w336:i16)
    }
    n111 = for {
      tunnel: w270 -> [w322] mode=indexing
      tunnel: [w323] -> w269 mode=indexing
      n112 = Unbundle By Name(w322) -> ("I"=w321:fxp<+/-,18,1>)
      n113 = To Fixed-Point(number=w321) -> (fixed-point=w320:fxp<+/-,16,1>)  [unwired: 1 in]
      n114 = Fixed-Point to Integer Cast(1:w320) -> (0:w323:i16)
    }
    n115 = for {
      tunnel: w295 -> [w348] mode=indexing
      tunnel: [w349] -> w294 mode=indexing
      n116 = Unbundle By Name(w348) -> ("I"=w347:fxp<+/-,18,1>)
      n117 = To Fixed-Point(number=w347) -> (fixed-point=w346:fxp<+/-,16,1>)  [unwired: 1 in]
      n118 = Fixed-Point to Integer Cast(1:w346) -> (0:w349:i16)
    }
    n119 = for {
      tunnel: w319 -> [w362] mode=indexing
      tunnel: [w361] -> w315 mode=indexing
      n120 = Unbundle By Name(w362) -> ("I"=w361:fxp<+/-,18,1>)
    }
    n121 = xnode ("High Throughput Multiply")("x"="ao.noise gain 3", "y"=w311, "input valid"=TRUE) -> ("x*y"=w318:fxp<+/-,41,5>[])  [unwired: 1 in, 2 out]
    n122 = xnode ("High Throughput Add")("x"=w315, "y"=w318, "input valid"=w316) -> ("x+y"=w310:fxp<+/-,16,1>[])  [unwired: 1 in, 2 out]
    n123 = for {
      tunnel: w310 -> [w360] mode=indexing
      tunnel: [w359] -> w279 mode=indexing
      n124 = Fixed-Point to Integer Cast(1:w360) -> (0:w359:i16)
    }
    n125 = Index Array(array=w294) -> (element #1=w293:i16, element #2=w292:i16)  [unwired: 2 in]
    n126 = Index Array(array=w289) -> (element #1=w290:i16, element #2=w291:i16)  [unwired: 2 in]
    n127 = Index Array(array=w269) -> (element #1=w268:i16, element #2=w267:i16)  [unwired: 2 in]
    n128 = Index Array(array=w279) -> (element #1=w266:i16, element #2=w265:i16)  [unwired: 2 in]
    n129 = xnode "FPGA I/O Node"("IO Module\\AO 1 Data N-1 Data Clock"=w290, "IO Module\\AO 1 Data N Data Clock"=w291) -> ()  [unwired: 2 in, 2 out]
    n130 = xnode "FPGA I/O Node"("IO Module\\AO 2 Data N-1 Data Clock"=w268, "IO Module\\AO 2 Data N Data Clock"=w267) -> ()  [unwired: 2 in, 2 out]
    n131 = xnode "FPGA I/O Node"("IO Module\\AO 3 Data N-1 Data Clock"=w266, "IO Module\\AO 3 Data N Data Clock"=w265) -> ()  [unwired: 2 in, 2 out]
    n132 = xnode "FPGA I/O Node"("IO Module\\AO 0 Data N-1 Data Clock"=w293, "IO Module\\AO 0 Data N Data Clock"=w292) -> ()  [unwired: 2 in, 2 out]
  }
  n133 = node-c288(w4) -> ()
